vi "Simple Reader.vi"(8 "error in (no error)":errorcluster, 11 "Simple VISA Reader Driver in":refnum<class "Simple VISA Reader Driver.lvclass">) -> (0 "error out":errorcluster, 1 "Signal names":string[](array[string]), 2 "Signals":dbl[](array[numeric]), 3 "Simple VISA Reader Driver out":refnum<class "Simple VISA Reader Driver.lvclass">, 4 "Signal units":string[](array[string]))   [LabVIEW 2015, in "Simple VISA Reader Driver.lvclass"]
uses:
  Simple VISA Reader Driver.lvclass
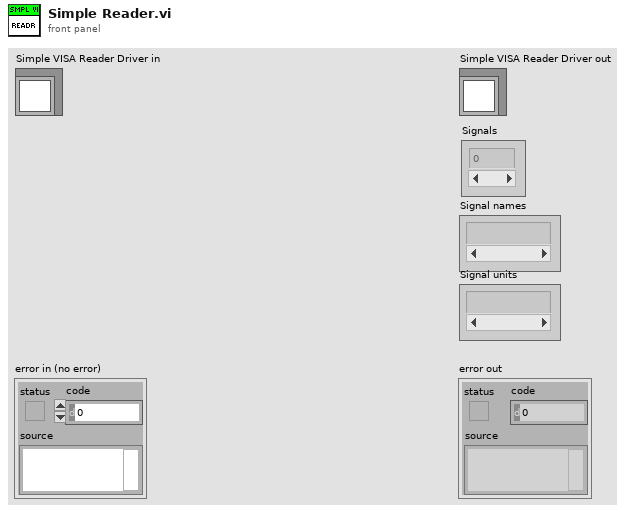
[diagram p1: front panel]
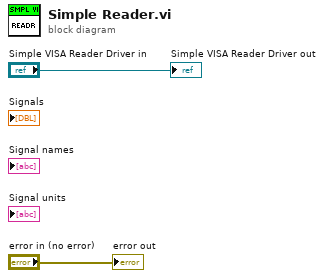
[diagram p0: block diagram]
diagram:
  "error out" <- "error in (no error)"
  "Simple VISA Reader Driver out" <- "Simple VISA Reader Driver in"
